vi "QMgr_DeQueue.vi"(7 "timeout in ms (-1)":i32=-1, 10 "error in (no error)":errorcluster, 11 "queue in":refnum<queue>) -> (2 "Command":string, 3 "queue out":refnum<queue>, 5 "data":variant)   [LabVIEW 2023, in "Jiaxin_Stepper_Controller.lvlib" / "MB Master.lvlib" / "MB_Master_TCP.lvclass"]
uses:
  MB_Master_TCP.lvclass
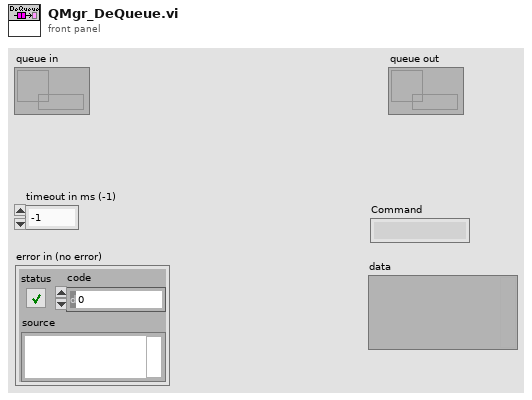
[diagram p1: front panel]
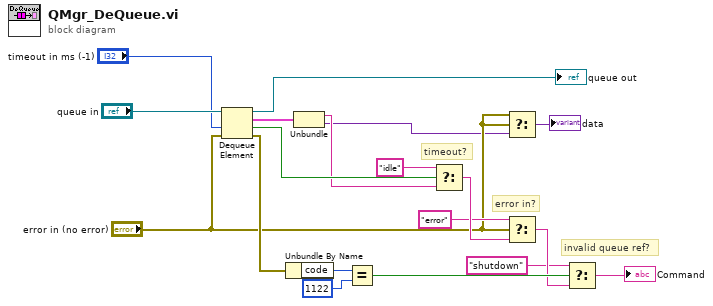
[diagram p0: block diagram]
diagram:
  # "timeout?"
  # "error in?"
  # "invalid queue ref?"
  n1 = Dequeue Element(queue="queue in", timeout in ms (-1)="timeout in ms (-1)", error in (no error)="error in (no error)") -> (queue out=→"queue out":refnum<queue>, element=w19:cluster{"cmd":string, "data":variant}, timed out?=w16:bool, error out=w10:errorcluster)
  n2 = Unbundle By Name(w10) -> ("code"=w9:i32)
  n3 = Unbundle(w19) -> ("cmd"=w15:string, "data"=w1:variant)
  n4 = Equal?(x=w9, y=1122) -> (x = y?=w7:bool)
  n5 = Select(t="idle", s=w16, f=w15) -> (s? t:f=w13:string)
  n6 = Select(t="error in (no error)", s="error in (no error)", f=w1) -> (s? t:f=→"data":variant)
  n7 = Select(t="error", s="error in (no error)", f=w13) -> (s? t:f=w6:string)
  n8 = Select(t="shutdown", s=w7, f=w6) -> (s? t:f=→"Command":string)
